vi "Creat RAW File.vi"(7 "#Cscan":dbl, 8 "error in":errorcluster, 10 "Scan Parameters":T1={"# Scan"={"#Ascan"=400, "#Bscan"=400}, "# Rpt"={"#ARpt"=1, "#BRpt"=1}, "Aline Rate"=2, "# Extra"={"# ARpt_extra"=5, "#Brtn_extra"=60}} {"Aline Rate" items=["76 KHz", "146 KHz", "76 KHz", "28 KHz", "10 KHz"]}, 11 "Save Path":path=path "E:/Jiarui/1217test") -> (0 "error out":errorcluster, 3 "refnum out":refnum<file>, 4 "Save Name":string, 6 "Scan Parameter":string)   [LabVIEW 2017]
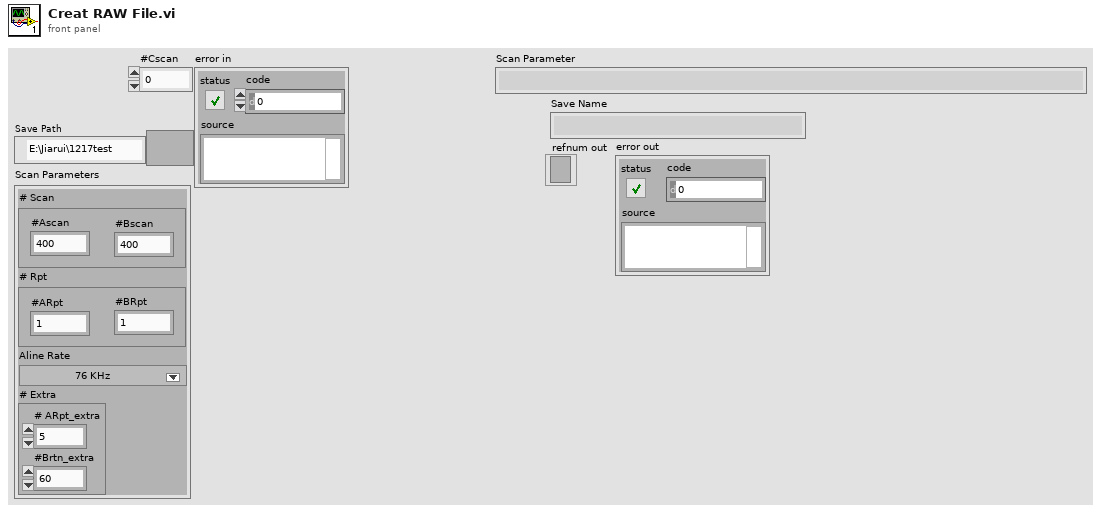
[diagram p1: front panel]
types:
  T1 = cluster{"# Scan":cluster{"#Ascan":i32, "#Bscan":i32}, "# Rpt":cluster{"#ARpt":i32, "#BRpt":i32}, "Aline Rate":u16, "# Extra":cluster{"# ARpt_extra":i32, "#Brtn_extra":i32}}
  T2 = enum16{"open", "replace", "create", "open or create", "replace or create", "replace or create with confirmation"}
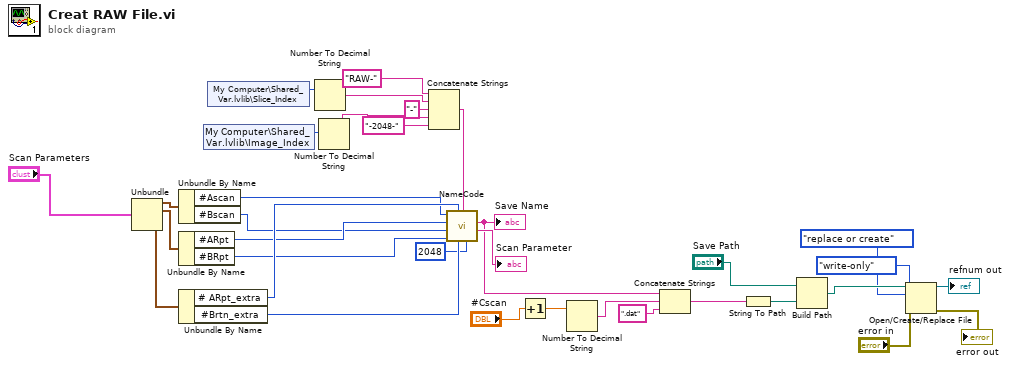
[diagram p0: block diagram]
diagram:
  n1 = Unbundle("Scan Parameters") -> ("# Scan"=w33:cluster{"#Ascan":i32, "#Bscan":i32}, "# Rpt"=w24:cluster{"#ARpt":i32, "#BRpt":i32}, "# Extra"=w23:cluster{"# ARpt_extra":i32, "#Brtn_extra":i32})  [unwired: 1 out]
  n2 = Unbundle By Name(w33) -> ("#Ascan"=w18:i32, "#Bscan"=w16:i32)
  n3 = Unbundle By Name(w24) -> ("#ARpt"=w17:i32, "#BRpt"=w15:i32)
  n4 = Unbundle By Name(w23) -> ("# ARpt_extra"=w22:i32, "#Brtn_extra"=w21:i32)
  n5 = shared-variable "My Computer\\Shared_Var.lvlib\\Image_Index"() -> (w28:i16)  [unwired: 1 in, 1 out]
  n6 = shared-variable "My Computer\\Shared_Var.lvlib\\Slice_Index"() -> (w31:i16)  [unwired: 1 in, 1 out]
  n7 = Number To Decimal String(number=w31) -> (decimal integer string=w30:string)  [unwired: 1 in]
  n8 = Number To Decimal String(number=w28) -> (decimal integer string=w27:string)  [unwired: 1 in]
  n9 = Concatenate Strings("RAW-" ("Name0"), w30, "-" ("string"), w27, "-2048-" ("string")) -> (w25:string)
  n10 = call "NameCode.vi"("# Z"=2048, "Name0"=w25, "# BRtn extra"=w21, "# ARpt extra"=w22, "# B rpt"=w15, "# B scan"=w16, "# A rpt"=w17, "# Aline"=w18) -> ("Scan Parameter"=→"Scan Parameter":string, "Name Code"=w9:string)  [unwired: 2 in]
  "Save Name" <- w9
  n11 = Increment(x="#Cscan") -> (x+1=w10:dbl)
  n12 = Number To Decimal String(number=w10) -> (decimal integer string=w11:string)  [unwired: 1 in]
  n13 = Concatenate Strings(w9, w11, ".dat" ("string")) -> (w13:string)
  n14 = String To Path(string=w13) -> (path=w14:path)
  n15 = Build Path(base path="Save Path", name or relative path=w14) -> (appended path=w6:path)
  n16 = Open/Create/Replace File(file path (use dialog)=w6, error in="error in", operation (0:open)=T2."replace or create", access (0:read/write)=enum16{"read/write", "read-only", "write-only"}."write-only") -> (refnum out=→"refnum out":refnum<file>, error out=→"error out":errorcluster)  [unwired: 2 in, 1 out]
